vi "Main Abstraction Level 6.vi"() -> ()   [LabVIEW 2023]
doc: "This is the complete measurement application, the result of all the design effort in the earlier Main Abstraction Level VIs."
uses:
  subVIs/Simulated Signal Type.ctl
  messages/MeasureAndLogMessage.lvclass/MeasureAndLogMessage.ctl
  subVIs/Measure and Log Settings.ctl
  <extravilib>/ChannelInstances/Stream-a[.](wfm(dbl))/EndpointRead.vi
  <vilib>/ChannelSupport/Channel Message/Read ID.vi
  <extravilib>/ChannelInstances/Stream-a[.](wfm(dbl))/Endpoint.vi
  <extravilib>/ChannelInstances/Stream-str/EndpointRead.vi
  <extravilib>/ChannelInstances/Lossy Stream-a[.](wfm(dbl))/EndpointRead.vi
  <extravilib>/ChannelInstances/Lossy Stream-a[.](wfm(dbl))/Endpoint.vi
  <extravilib>/ChannelInstances/Stream-str/Endpoint.vi
  messages/MeasureAndLogMessage.lvclass
  c:/dev/_r/4/eng/lv-core/lvpostprocessingd/lv_mc_x86_64/dist_i386/vi.lib/ChannelSupport/Channel Message/Channel Message.lvclass
  <extravilib>/ChannelInstances/Tag-path/Instantiate.vi
  <extravilib>/ChannelInstances/Stream-a[.](wfm(dbl))/Instantiate.vi
  <extravilib>/ChannelInstances/Stream-a[.](wfm(dbl))/)Channel.vi
  <resource>/ChannelSupport/_ChannelSupport/WaitIfNeeded.vi
  <extravilib>/ChannelInstances/Tag-path/EndpointRead.vi
  <vilib>/Waveform/WDTFileIO.llb/Write Waveforms to File (1D).vi
  <extravilib>/ChannelInstances/Lossy Stream-a[.](wfm(dbl))/Instantiate.vi
  <extravilib>/ChannelInstances/Lossy Stream-a[.](wfm(dbl))/)Channel.vi
  <extravilib>/ChannelInstances/Messenger-class'MeasureAndLogMessage'/Instantiate.vi
  <extravilib>/ChannelInstances/Messenger-class'MeasureAndLogMessage'/Endpoint.vi
  <extravilib>/ChannelInstances/Stream-str/Instantiate.vi
  <extravilib>/ChannelInstances/Stream-str/)Channel.vi
  <extravilib>/ChannelInstances/Tag-bool/Instantiate.vi
  <extravilib>/ChannelInstances/Tag-t'Measure and Log Settings.ctl'/Instantiate.vi
  <extravilib>/ChannelInstances/Tag-t'Measure and Log Settings.ctl'/Endpoint.vi
  <extravilib>/ChannelInstances/Tag-path/Endpoint.vi
  <extravilib>/ChannelInstances/Tag-bool/Endpoint.vi
  <extravilib>/ChannelInstances/Tag-bool/EndpointRead.vi
  <extravilib>/ChannelInstances/Tag-t'Measure and Log Settings.ctl'/EndpointRead.vi
  <extravilib>/ChannelInstances/Stream-str.lvlib
  <extravilib>/ChannelInstances/Lossy Stream-a[.](wfm(dbl)).lvlib
  <extravilib>/ChannelInstances/Tag-bool.lvlib
  <extravilib>/ChannelInstances/Stream-a[.](wfm(dbl)).lvlib
  <extravilib>/ChannelInstances/Tag-path.lvlib
  <extravilib>/ChannelInstances/Tag-t'Measure and Log Settings.ctl'.lvlib
  <extravilib>/ChannelInstances/Messenger-class'MeasureAndLogMessage'.lvlib
panel:
  in  "Exit flag":bool
  in  "Record":bool
  in  "Stop":bool
  out "Data":waveform(dbl)[](graph)
  out "Status":string
  in  "Settings":bool
  in  "Start":bool
  in  "Exit":bool
  # "Continuous Measurement Data Logger"
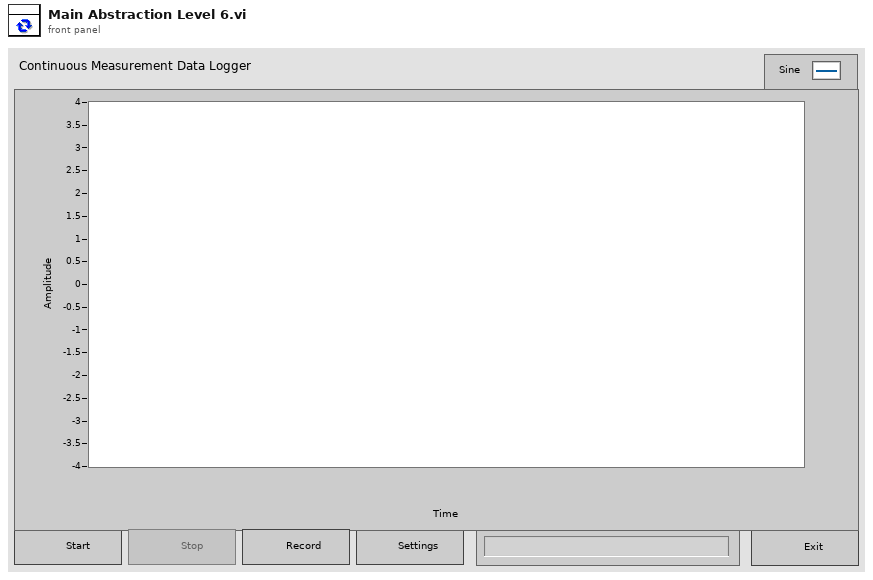
[diagram p1: front panel]
types:
  T1 = typedef "Measure and Log Settings.ctl" = cluster{"sample rate":dbl, "input range":dbl, "logfile path":path, "Simulated Signal":cluster{"signal type":T2, "frequency":dbl, "amplitude":dbl}}
  T2 = typedef "Simulated Signal Type.ctl" = enum16{"Sine Wave", "Square Wave with Noise"}
  T3 = enum8{"Enabled", "Disabled", "Disabled and Grayed Out"}
  T4 = typedef "Messenger-class'MeasureAndLogMessage'.lvlib/))Channel.ctl" = refnum<queue>
  T5 = typedef "Tag-t'Measure and Log Settings.ctl'.lvlib/))Channel.ctl" = refnum<queue>
  T6 = typedef "Tag-path.lvlib/))Channel.ctl" = refnum<queue>
  T7 = typedef "Tag-bool.lvlib/))Channel.ctl" = refnum<queue>
  T8 = typedef "Stream-a[.](wfm(dbl)).lvlib/)Channel.ctl" = refnum<queue>
  T9 = typedef "Stream-str.lvlib/)Channel.ctl" = refnum<queue>
  T10 = typedef "Lossy Stream-a[.](wfm(dbl)).lvlib/)Channel.ctl" = refnum<queue>
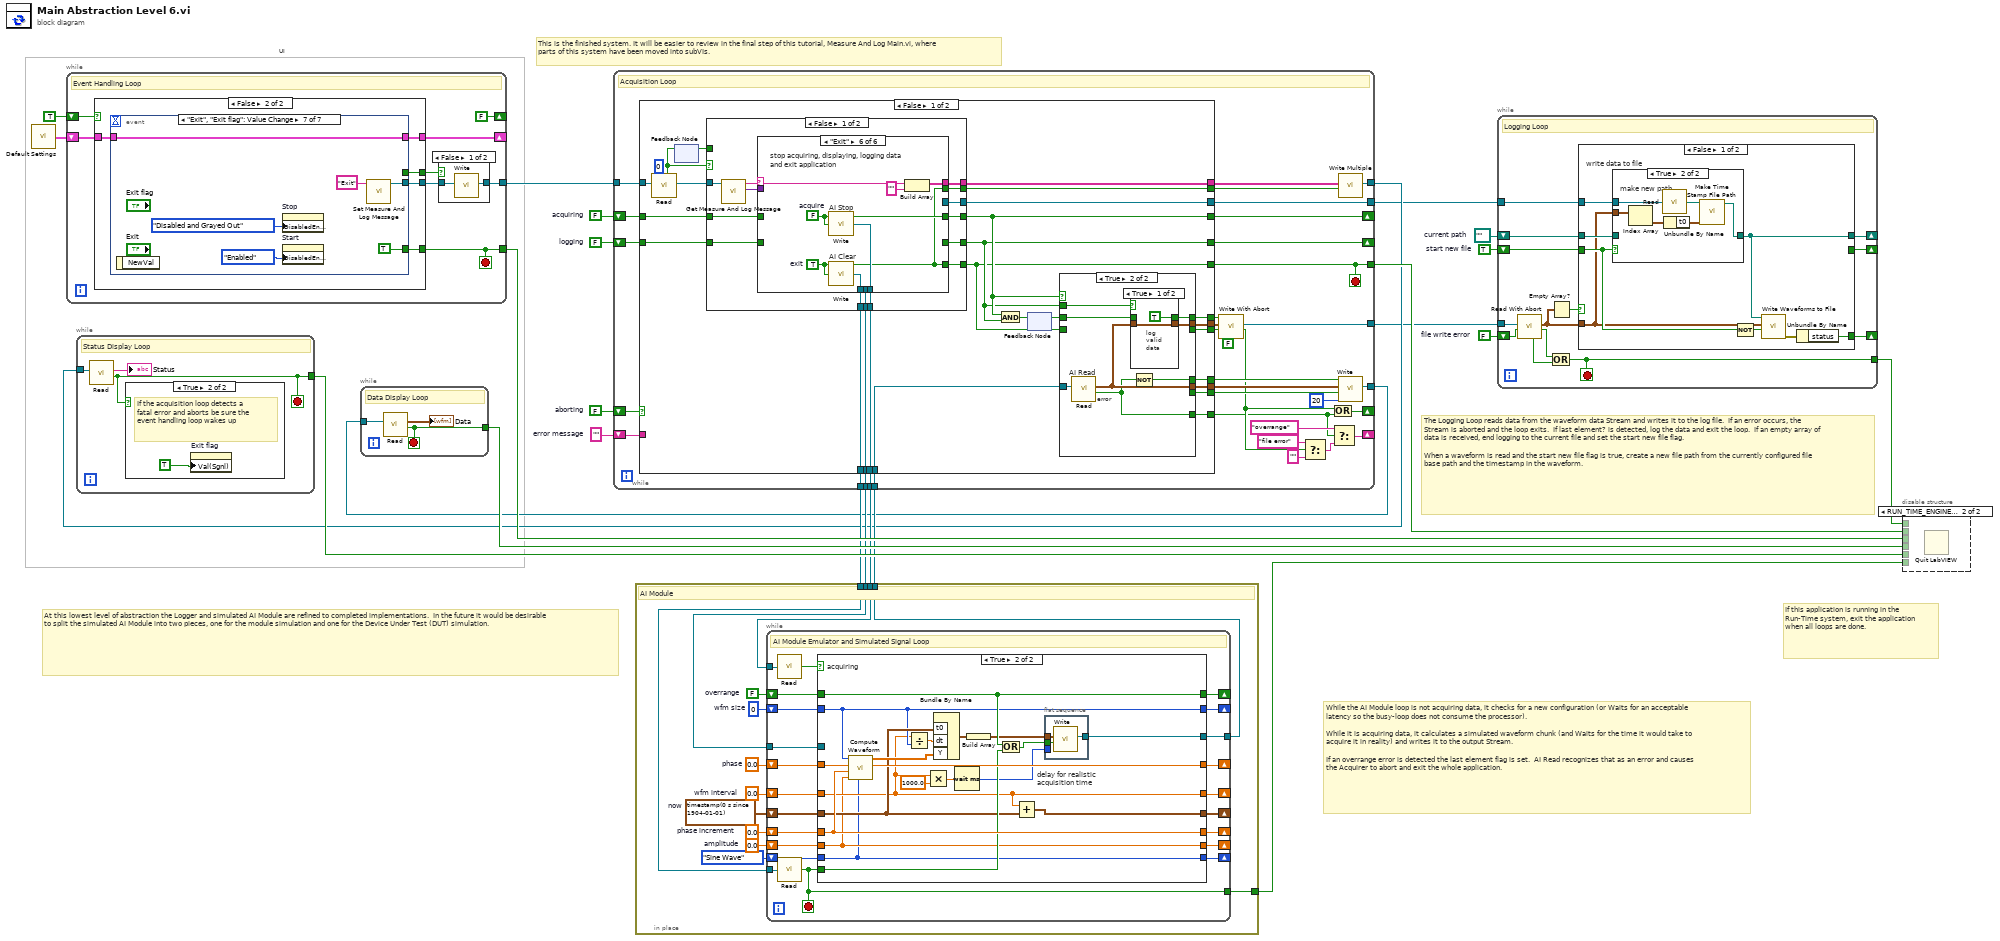
[diagram p0: block diagram]
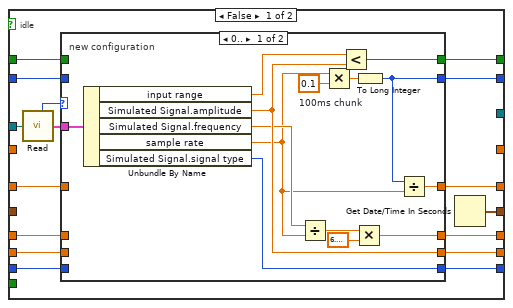
[diagram p2: hidden frame]
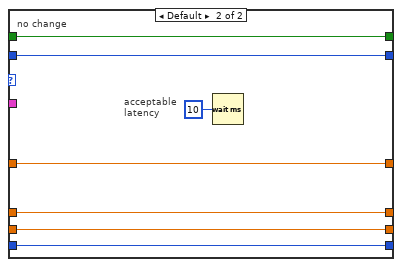
[diagram p3: hidden frame]
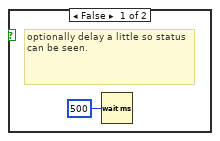
[diagram p4: hidden frame]
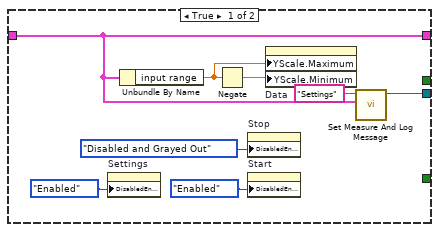
[diagram p5: hidden frame]
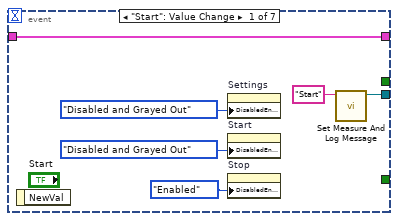
[diagram p6: hidden frame]
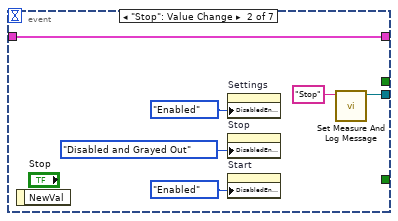
[diagram p7: hidden frame]
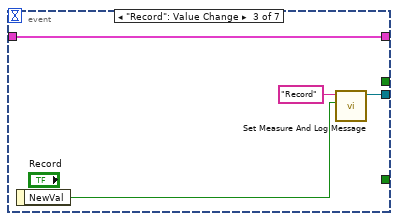
[diagram p8: hidden frame]
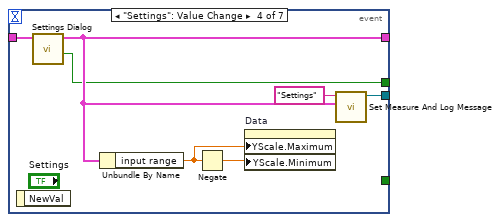
[diagram p9: hidden frame]
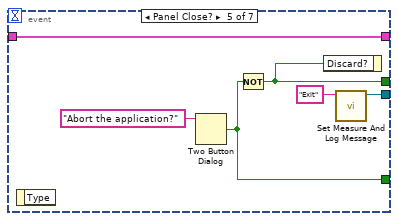
[diagram p10: hidden frame]
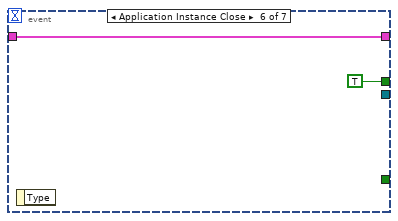
[diagram p11: hidden frame]
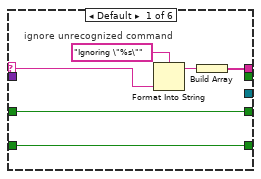
[diagram p14: hidden frame]
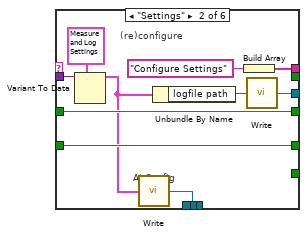
[diagram p15: hidden frame]
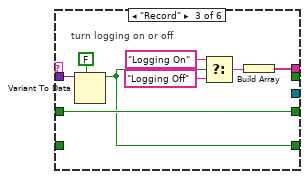
[diagram p16: hidden frame]
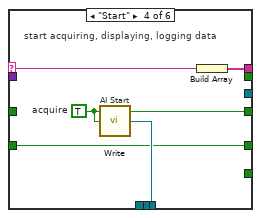
[diagram p17: hidden frame]
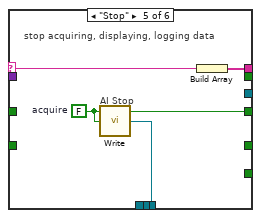
[diagram p18: hidden frame]
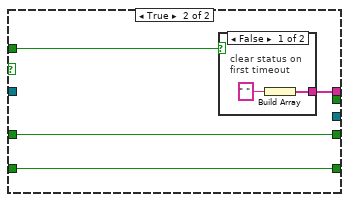
[diagram p19: hidden frame]
diagram:
  w2 = ""  # error message
  w4 = FALSE  # file write error
  w5 = path ""  # current path
  w6 = TRUE  # start new file
  w8 = FALSE  # aborting
  w10 = FALSE  # logging
  w11 = FALSE  # acquiring
  # "This is the finished system. It will be easier to review in the final step of this tutorial, Measure And Log Main.vi, where parts of this system have been moved into subVIs."
  # "At this lowest level of abstraction the Logger and simulated AI Module are refined to completed implementations.  In the future it would be desirable to split the simulated AI Module into two pieces, one for the module simulation and one for the Device Under Test (DUT) simulation."
  # "If this application is running in the Run-Time system, exit the application when all loops are done."
  # "The Logging Loop reads data from the waveform data Stream and writes it to the log file.  If an error occurs, the Stream is aborted and the loop exits.  If last element? is detected, log the data and exit the loop.  If an empty array of data is received, end logging to the current file and set the start new file flag.\n\nWhen a waveform is read and the start new file flag is true, create a new file path from the currently configured file base path and the timestamp in the waveform."
  # "While the AI Module loop is not acquiring data, it checks for a new configuration (or Waits for an acceptable latency so the busy-loop does not consume the processor).\n\nWhile it is acquiring data, it calculates a simulated waveform chunk (and Waits for the time it would take to acquire it in reality) and writes it to the output Stream.\n\nIf an overrange error is detected the last element flag is set.  AI Read recognizes that as an error and causes the Acquirer to abort and exit the whole application."
  # "UI"
  n1 = call "Default Settings.vi"() -> ("default settings"=w7:T1)
  n2 = while {
    tunnel: [w29] -> w14
    tunnel: [w32] -> w24
    shift-right: [w31] -> _
    shift-left: w7 -> [w30]
    shift-right: [FALSE] -> _
    shift-left: TRUE -> [w26]
    stop <- w32 stop-if-true
    # "Event Handling Loop"
    n3 = case shown="False" w26 {
      tunnel: [_ w45] -> w32
      tunnel: [w39 w44] -> w31
      tunnel: w30 -> [w39 w43]
      tunnel: [w35 w42] -> w28
      tunnel: [_ w41] -> w27
      frame True {
        n4 = property on="Settings" class="Bool"("DisabledEnum"=T3."Enabled" ("Disabled")) -> ()  [unwired: 2 in, 2 out]
        n5 = Unbundle By Name(w39) -> ("input range"=w33:dbl)
        n6 = Negate(x=w33) -> (-x=w34:dbl)
        n7 = property on="Stop" class="Bool"("DisabledEnum"=T3."Disabled and Grayed Out" ("Disabled")) -> ()  [unwired: 2 in, 2 out]
        n8 = property on="Start" class="Bool"("DisabledEnum"=T3."Enabled" ("Disabled")) -> ()  [unwired: 2 in, 2 out]
        n9 = property on="Data" class="WFChart (strict)"("YScale.Maximum"=w33, "YScale.Minimum"=w34) -> ()  [unwired: 2 in, 2 out]
        n10 = call "Set Measure And Log Message.vi"("args"=w39, "command"="Settings") -> ("MyMessage"=w35:refnum<class "MeasureAndLogMessage.lvclass">)  [unwired: 9 in]
      }
      frame False {
        n11 = event shown="[6] \"Exit\", \"Exit flag\": Value Change" {
          selector: _ -> [_ _ _ _ _ _ _]
          dyn-events: _ -> [_ _ _ _ _ _ _]
          timeout: _ -> [_ _ _ _ _ _ _]
          tunnel: [_ _ _ _ w70 _ TRUE] -> w45
          tunnel: [w47 w53 w59 w67 w73 w76 w78] -> w44
          tunnel: w43 -> [w47 w53 w59 w68 w73 w76 w78]
          tunnel: [w46 w52 w58 w66 w71 _ w77] -> w42
          tunnel: [_ _ _ w64 w69 TRUE ("cancelled") _] -> w41
          event "Start": Value Change {
            n12 = event-data() -> ()  [unwired: 1 in, 1 out]
            n13 = property on="Settings" class="Bool"("DisabledEnum"=T3."Disabled and Grayed Out" ("Disabled")) -> ()  [unwired: 2 in, 2 out]
            n14 = property on="Start" class="Bool"("DisabledEnum"=T3."Disabled and Grayed Out" ("Disabled")) -> ()  [unwired: 2 in, 2 out]
            n15 = property on="Stop" class="Bool"("DisabledEnum"=T3."Enabled" ("Disabled")) -> ()  [unwired: 2 in, 2 out]
            n16 = call "Set Measure And Log Message.vi"("command"="Start") -> ("MyMessage"=w46:refnum<class "MeasureAndLogMessage.lvclass">)  [unwired: 10 in]
          }
          event "Stop": Value Change {
            n17 = event-data() -> ()  [unwired: 1 in, 1 out]
            n18 = property on="Settings" class="Bool"("DisabledEnum"=T3."Enabled" ("Disabled")) -> ()  [unwired: 2 in, 2 out]
            n19 = property on="Stop" class="Bool"("DisabledEnum"=T3."Disabled and Grayed Out" ("Disabled")) -> ()  [unwired: 2 in, 2 out]
            n20 = property on="Start" class="Bool"("DisabledEnum"=T3."Enabled" ("Disabled")) -> ()  [unwired: 2 in, 2 out]
            n21 = call "Set Measure And Log Message.vi"("command"="Stop") -> ("MyMessage"=w52:refnum<class "MeasureAndLogMessage.lvclass">)  [unwired: 10 in]
          }
          event "Record": Value Change {
            n22 = event-data() -> ("NewVal"=w60:bool)  [unwired: 1 in]
            n23 = call "Set Measure And Log Message.vi"("args"=w60, "command"="Record") -> ("MyMessage"=w58:refnum<class "MeasureAndLogMessage.lvclass">)  [unwired: 9 in]
          }
          event "Settings": Value Change {
            n24 = event-data() -> ()  [unwired: 1 in, 1 out]
            n25 = call "Settings Dialog.vi"("settings in"=w68) -> ("cancelled"=w64:bool, "settings out"=w67:T1)  [unwired: 9 in]
            n26 = Unbundle By Name(w67) -> ("input range"=w62:dbl)
            n27 = Negate(x=w62) -> (-x=w63:dbl)
            n28 = property on="Data" class="WFChart (strict)"("YScale.Maximum"=w62, "YScale.Minimum"=w63) -> ()  [unwired: 2 in, 2 out]
            n29 = call "Set Measure And Log Message.vi"("args"=w67, "command"="Settings") -> ("MyMessage"=w66:refnum<class "MeasureAndLogMessage.lvclass">)  [unwired: 9 in]
          }
          event Panel Close? {
            n30 = event-data() -> ()  [unwired: 1 in, 1 out]
            n31 = Two Button Dialog(message="Abort the application?") -> (T button?=w70:bool)  [unwired: 2 in]
            n32 = Not(x=w70) -> (.not. x?=w69:bool)
            n33 = event-data("Discard?"=w69) -> ()  [unwired: 1 in, 1 out]
            n34 = call "Set Measure And Log Message.vi"("command"="Exit") -> ("MyMessage"=w71:refnum<class "MeasureAndLogMessage.lvclass">)  [unwired: 10 in]
          }
          event Application Instance Close {
            n35 = event-data() -> ()  [unwired: 1 in, 1 out]
          }
          event "Exit", "Exit flag": Value Change {
            n36 = event-data() -> ()  [unwired: 1 in, 1 out]
            n37 = property on="Stop" class="Bool"("DisabledEnum"=T3."Disabled and Grayed Out" ("Disabled")) -> ()  [unwired: 2 in, 2 out]
            n38 = property on="Start" class="Bool"("DisabledEnum"=T3."Enabled" ("Disabled")) -> ()  [unwired: 2 in, 2 out]
            n39 = call "Set Measure And Log Message.vi"("command"="Exit") -> ("MyMessage"=w77:refnum<class "MeasureAndLogMessage.lvclass">)  [unwired: 10 in]
          }
        }
      }
    }
    n40 = case shown="False" w27 {
      tunnel: [w84 _] -> w29
      tunnel: w28 -> [w83 _]
      frame False {
        n41 = call <extravilib>:"Write.vi"("element"=w83) -> ("channel"=w84:T4)  [unwired: 8 in, 2 out]
      }
      frame True {
      }
    }
  }
  n42 = while {
    tunnel: w15 -> [w87]
    tunnel: [w85] -> w23
    stop <- w85 stop-if-true
    # "Status Display Loop"
    n43 = call <extravilib>:"Read.vi"("channel"=w87) -> ("last element?"=w85:bool, "element"=→"Status":string)  [unwired: 6 in, 3 out]
    n44 = case shown="True" w85 {
      frame False {
        # "optionally delay a little so status can be seen."
        n45 = Wait (ms)(milliseconds to wait=u32 500) -> ()  [unwired: 1 out]
      }
      frame True {
        # "If the acquisition loop detects a fatal error and aborts be sure the event handling loop wakes up"
        n46 = property on="Exit flag" class="Bool (strict)"("Val(Sgnl)"=TRUE) -> ()  [unwired: 2 in, 2 out]
      }
    }
  }
  n47 = while {
    tunnel: [w92] -> w22
    tunnel: w13 -> [w90]
    stop <- w92 stop-if-true
    # "Data Display Loop"
    n48 = call <extravilib>:"Read.vi"("channel"=w90) -> ("last element?"=w92:bool, "element"=→"Data":waveform(dbl)[])  [unwired: 5 in, 4 out]
  }
  n49 = while {
    tunnel: w14 -> [w125]
    tunnel: [w113] -> w15
    tunnel: [w110] -> w13
    tunnel: [w106] -> w12
    tunnel: [w121] -> w18
    tunnel: w19 -> [w124]
    shift-right: [w118] -> _
    shift-left: w11 -> [w119]
    shift-right: [w117] -> _
    shift-left: w10 -> [w126]
    tunnel: [w123] -> w9
    tunnel: [w122] -> w17
    tunnel: [w120] -> w16
    shift-right: [w105] -> _
    shift-left: w8 -> [w116]
    shift-right: [w96] -> _
    shift-left: w2 -> [w115]
    tunnel: [w114] -> w21
    stop <- w114 stop-if-true
    # "Acquisition Loop"
    n50 = case shown="False" w116 {
      tunnel: w126 -> [w152 _]
      tunnel: w125 -> [w151 _]
      tunnel: w124 -> [w149 _]
      tunnel: [w145 _] -> w123
      tunnel: [w144 _] -> w122
      tunnel: [w143 w231] -> w121
      tunnel: [w142 w230] -> w120
      tunnel: w119 -> [w141 _]
      tunnel: [w140 w232] -> w118
      tunnel: [w139 _] -> w117
      tunnel: [w136 w227] -> w114
      tunnel: w115 -> [_ w229]
      tunnel: [w134 w227] -> w112
      tunnel: [w135 w228] -> w111
      tunnel: [w132 w227] -> w109
      tunnel: [w133 _] -> w108
      tunnel: [w131 _] -> w107
      tunnel: [w130 _] -> w97
      tunnel: [w129 _] -> w104
      tunnel: [w128 w227] -> w103
      tunnel: [w127 _] -> w102
      frame False {
        n51 = call <extravilib>:"Read.vi"("timeout in ms (-1)"=0, "channel"=w151) -> ("element"=w150:refnum<class "MeasureAndLogMessage.lvclass">, "timed out?"=w147:bool)  [unwired: 7 in, 1 out]
        n52 = feedback #1() -> (w146:bool)  [unwired: 1 in]
        n53 = feedback-in #1(w147) -> ()
        n54 = case shown="False" w147 {
          tunnel: w150 -> [w166 _]
          tunnel: [w162 _] -> w143
          tunnel: [w163 _] -> w136
          tunnel: [w161 w210] -> w140
          tunnel: w141 -> [w160 w210]
          tunnel: [w159 w209] -> w139
          tunnel: w152 -> [w158 w209]
          tunnel: w146 -> [_ w208]
          tunnel: [w157 _] -> w145
          tunnel: [w156 _] -> w144
          tunnel: [w155 _] -> w142
          tunnel: [w154 w207] -> w135
          tunnel: [w153 _] -> w134
          frame False {
            n55 = call "Get Measure And Log Message.vi"("MyMessage"=w166) -> ("args"=w164:variant, "command"=w165:string)  [unwired: 7 in, 2 out]
            n56 = case shown="\"Exit\"" w165 {
              selector: w165 -> [w172 _ _ w192 w197 w206]
              tunnel: w164 -> [_ w180 w189 _ _ _]
              tunnel: [_ _ _ w195 w199 w203] -> w162
              tunnel: [_ _ _ _ _ w200] -> w163
              tunnel: [w170 w182 w190 w194 w198 w204] -> w161
              tunnel: w160 -> [w170 w182 w190 _ _ _]
              tunnel: [w169 w181 w185 w193 _ _] -> w159
              tunnel: w158 -> [w169 w181 _ w193 _ _]
              tunnel: [_ w177 _ _ _ _] -> w157
              tunnel: [_ w176 _ _ _ _] -> w156
              tunnel: [_ _ _ _ _ w202] -> w155
              tunnel: [w167 w173 w183 w191 w196 w201] -> w154
              tunnel: [_ _ _ _ _ w200] -> w153
              frame Default {
                # "ignore unrecognized command"
                n57 = Format Into String(format string="Ignoring \"%s\"", w172) -> (resulting string=w168:string)  [unwired: 2 in, 1 out]
                n58 = Build Array(w168) -> (w167:string[])
              }
              frame "Settings" {
                # "AI Config"
                # "(re)configure"
                n59 = Variant To Data(type=T1 {"sample rate"=100.0, "input range"=10.0, "logfile path"=path "/Bohr/Users/jeffk/Documents/LabVIEW Data/Logged Data.tdms", "Simulated Signal"={"signal type"=enum."Sine Wave", "frequency"=1000.0, "amplitude"=5.0}} ("settings out"), Variant=w180) -> (data=w179:T1)  [unwired: 1 in, 1 out]
                n60 = call <extravilib>:"Write.vi"("element"=w179) -> ("channel"=w176:T5)  [unwired: 1 out]
                n61 = Unbundle By Name(w179) -> ("logfile path"=w178:path)
                n62 = Build Array("Configure Settings" ("element")) -> (w173:string[])
                n63 = call <extravilib>:"Write.vi"("element"=w178) -> ("channel"=w177:T6)  [unwired: 1 out]
              }
              frame "Record" {
                # "turn logging on or off"
                n64 = Variant To Data(type=FALSE, Variant=w189) -> (data=w185:bool)  [unwired: 1 in, 1 out]
                n65 = Select(t="Logging On", s=w185, f="Logging Off") -> (s? t:f=w184:string)
                n66 = Build Array(w184) -> (w183:string[])
              }
              frame "Start" {
                w194 = TRUE  # acquire
                # "AI Start"
                # "start acquiring, displaying, logging data"
                n67 = call <extravilib>:"Write.vi"("element"=w194) -> ("channel"=w195:T7)  [unwired: 1 out]
                n68 = Build Array(w192) -> (w191:string[])
              }
              frame "Stop" {
                w198 = FALSE  # acquire
                # "AI Stop"
                # "stop acquiring, displaying, logging data"
                n69 = call <extravilib>:"Write.vi"("element"=w198) -> ("channel"=w199:T7)  [unwired: 1 out]
                n70 = Build Array(w197) -> (w196:string[])
              }
              frame "Exit" {
                w204 = FALSE  # acquire
                w200 = TRUE  # exit
                # "AI Clear"
                # "AI Stop"
                # "stop acquiring, displaying, logging data\nand exit application"
                n71 = call <extravilib>:"Write.vi"("element"=w204) -> ("channel"=w203:T7)  [unwired: 1 out]
                n72 = call <extravilib>:"Write.vi"("element"=w200) -> ("channel"=w202:T7)  [unwired: 1 out]
                n73 = Build Array(w206, "" ("element")) -> (w201:string[])
              }
            }
          }
          frame True {
            n74 = case shown="False" w208 {
              tunnel: [w211 _] -> w207
              frame False {
                # "clear status on\nfirst timeout"
                n75 = Build Array(" " ("string")) -> (w211:string[])
              }
              frame True {
              }
            }
          }
        }
        n76 = And(x=w140, y=w139) -> (x .and. y?=w138:bool)
        n77 = feedback #2() -> (w137:bool)  [unwired: 1 in]
        n78 = feedback-in #2(w138) -> ()
        n79 = case shown="True" w140 {
          tunnel: w149 -> [_ w223]
          tunnel: w139 -> [_ w222]
          tunnel: w137 -> [w215 w221]
          tunnel: w136 -> [w214 _]
          tunnel: [_ w219] -> w133
          tunnel: [w214 _] -> w132
          tunnel: [_ w220] -> w131
          tunnel: [_ w216] -> w130
          tunnel: [w215 w217] -> w129
          tunnel: [w214 _] -> w128
          tunnel: [_ w218] -> w127
          frame False {
            # "acceptable\nlatency"
            n80 = Wait (ms)(milliseconds to wait=u32 30) -> ()  [unwired: 1 out]
          }
          frame True {
            # "error"
            # "AI Read"
            n81 = call <extravilib>:"Read.vi"("channel"=w223) -> ("last element?"=w216:bool, "element"=w220:waveform(dbl)[])  [unwired: 6 in, 3 out]
            n82 = case shown="True" w222 {
              tunnel: w220 -> [w225 _]
              tunnel: w221 -> [_ w226]
              tunnel: [w225 _] -> w218
              tunnel: [TRUE w226] -> w217
              frame True {
                # "log \nvalid\ndata"
              }
              frame False {
              }
            }
            n83 = Not(x=w216) -> (.not. x?=w219:bool)
          }
        }
      }
      frame True {
        w232 = FALSE  # acquire
        w227 = TRUE  # exit
        # "aborting due to AI or file error"
        # "AI Clear"
        # "AI Stop"
        # "stop acquiring, displaying, logging data\nand exit application with error message"
        n84 = call <extravilib>:"Write.vi"("element"=w232) -> ("channel"=w231:T7)  [unwired: 1 out]
        n85 = call <extravilib>:"Write.vi"("element"=w227) -> ("channel"=w230:T7)  [unwired: 1 out]
        n86 = Build Array(w229) -> (w228:string[])
      }
    }
    n87 = call <extravilib>:"Write With Abort.vi"("abort"=FALSE, "last element? (F)"=w103, "element"=w102, "element valid? (T)"=w104) -> ("aborted?"=w100:bool, "channel"=w106:T8)  [unwired: 4 in, 2 out]
    n88 = Select(t="file error", s=w100, f="") -> (s? t:f=w95:string)
    n89 = Or(x=w100, y=w97) -> (x .or. y?=w105:bool)
    n90 = Select(t="overrange", s=w97, f=w95) -> (s? t:f=w96:string)
    n91 = call <extravilib>:"Write Multiple.vi"("last element? (F)"=w112, "elements"=w111) -> ("channel"=w113:T9)  [unwired: 6 in, 3 out]
    n92 = call <extravilib>:"Write.vi"("size (1)"=20, "last element? (F)"=w109, "element"=w107, "element valid? (T)"=w108) -> ("channel"=w110:T10)  [unwired: 5 in, 2 out]
  }
  n93 = in-place {
    in-place-border: [w243] -> w19
    in-place-border: w18 -> [w242]
    in-place-border: w17 -> [w241]
    in-place-border: w16 -> [w240]
    in-place-border: [w233] -> w20
    w235 = timestamp(0 s since 1904-01-01)  # now
    w236 = 0.0  # wfm interval
    w237 = 0  # wfm size
    w238 = FALSE  # overrange
    w239 = 0.0  # amplitude
    w245 = 0.0  # phase increment
    w244 = 0.0  # phase
    # "AI Module"
    n94 = while {
      shift-right: [w266] -> _
      shift-left: w244 -> [w267]
      tunnel: [w265] -> w243
      tunnel: w242 -> [w262]
      tunnel: w240 -> [w261]
      tunnel: w241 -> [w260]
      shift-right: [w259] -> _
      shift-left: w245 -> [w264]
      shift-right: [w258] -> _
      shift-left: Simulated_Signal_Type."Sine Wave" ("signal type") -> [w257]
      shift-right: [w256] -> _
      shift-left: w239 -> [w255]
      shift-right: [w254] -> _
      shift-left: w238 -> [w253]
      shift-right: [w252] -> _
      shift-left: w237 -> [w251]
      shift-right: [w250] -> _
      shift-left: w236 -> [w248]
      shift-right: [w249] -> _
      shift-left: w235 -> [w247]
      tunnel: [w246] -> w233
      stop <- w246 stop-if-true
      # "AI Module Emulator and Simulated Signal Loop"
      n95 = call <extravilib>:"Read.vi"("channel"=w262) -> ("element"=w263:bool)  [unwired: 1 in, 1 out]
      n96 = call <extravilib>:"Read.vi"("channel"=w261) -> ("element"=w246:bool)  [unwired: 1 in, 1 out]
      n97 = case shown="True" w263 {
        tunnel: w267 -> [_ w324]
        tunnel: [_ w323] -> w266
        tunnel: [_ w312] -> w265
        tunnel: w264 -> [w283 w322]
        tunnel: w246 -> [_ w320]
        tunnel: w260 -> [w270 _]
        tunnel: [w282 w322] -> w259
        tunnel: [w281 w306] -> w258
        tunnel: w257 -> [w280 w306]
        tunnel: [w279 w307] -> w256
        tunnel: w255 -> [w278 w307]
        tunnel: [w277 w321] -> w254
        tunnel: w253 -> [w276 w321]
        tunnel: [w275 w315] -> w252
        tunnel: w251 -> [w274 w315]
        tunnel: [w273 w311] -> w250
        tunnel: [w272 w319] -> w249
        tunnel: w248 -> [w271 w311]
        tunnel: w247 -> [_ w317]
        frame False {
          # "idle"
          n98 = call <extravilib>:"Read.vi"("channel"=w270) -> ("missed"=w269:i32, "element"=w268:T1)  [unwired: 1 in]
          n99 = case shown="0.." w269 {
            tunnel: w268 -> [w297 _]
            tunnel: w283 -> [_ w304]
            tunnel: [w290 w304] -> w282
            tunnel: [w295 w303] -> w281
            tunnel: w280 -> [_ w303]
            tunnel: [w292 w302] -> w279
            tunnel: w278 -> [_ w302]
            tunnel: [w294 w301] -> w277
            tunnel: w276 -> [_ w301]
            tunnel: [w286 w300] -> w275
            tunnel: w274 -> [_ w300]
            tunnel: [w285 w299] -> w273
            tunnel: w271 -> [_ w299]
            frame 0.. {
              w289 = 0.1  # 100ms chunk
              # "new configuration"
              n100 = Unbundle By Name(w297) -> ("input range"=w293:dbl, "Simulated Signal.amplitude"=w292:dbl, "Simulated Signal.frequency"=w287:dbl, "sample rate"=w284:dbl, "Simulated Signal.signal type"=w295:T2)
              n101 = Divide(x=w287, y=w284) -> (x/y=w291:dbl)
              n102 = Multiply(x=w284, y=w289) -> (x*y=w288:dbl)
              n103 = Less?(x=w293, y=w292) -> (x < y?=w294:bool)
              n104 = Multiply(x=w291, y=6.283185307179586) -> (x*y=w290:dbl)
              n105 = To Long Integer(number=w288) -> (32bit integer=w286:i32)
              n106 = Divide(x=w286, y=w284) -> (x/y=w285:dbl)
            }
            frame Default {
              # "acceptable\nlatency"
              # "no change"
              n107 = Wait (ms)(milliseconds to wait=u32 10) -> ()  [unwired: 1 out]
            }
          }
          n108 = Get Date/Time In Seconds() -> (seconds since 1Jan1904=w272:timestamp)
        }
        frame True {
          # "delay for realistic\nacquisition time"
          # "acquiring"
          n109 = call "Compute Waveform.vi"("signal type"=w306, "amplitude"=w307, "phase increment"=w322, "phase in"=w324, "wfm size"=w315) -> ("phase out"=w323:dbl, "wfm array"=w318:dbl[])  [unwired: 5 in]
          n110 = Divide(x=w311, y=w315) -> (x/y=w316:dbl)
          n111 = Multiply(x=w311, y=1000.0) -> (x*y=w309:dbl)
          n112 = Bundle By Name("t0"=w317, "dt"=w316, "Y"=w318) -> (w314:waveform(dbl))  [unwired: 1 in]
          n113 = Wait (ms)(milliseconds to wait=w309) -> (millisecond timer value=w305:u32)
          n114 = Build Array(w314) -> (w313:waveform(dbl)[])
          n115 = Or(x=w321, y=w320) -> (x .or. y?=w308:bool)
          n116 = Add(x=w311, y=w317) -> (x+y=w319:timestamp)
          n117 = flat-sequence {
            tunnel: w313 -> [w327]
            tunnel: [w326] -> w312
            tunnel: w308 -> [w325]
            tunnel: w305 -> [_]
            frame #0 {
              n118 = call <extravilib>:"Write.vi"("last element? (F)"=w325, "element"=w327) -> ("channel"=w326:T8)  [unwired: 7 in, 2 out]
            }
          }
        }
      }
    }
  }
  n119 = while {
    tunnel: w12 -> [w340]
    tunnel: w9 -> [w335]
    shift-right: [w337] -> _
    shift-left: w6 -> [w336]
    shift-right: [w334] -> _
    shift-left: w5 -> [w333]
    shift-right: [w331] -> _
    shift-left: w4 -> [w330]
    tunnel: [w328] -> w3
    stop <- w328 stop-if-true
    # "Logging Loop"
    n120 = call <extravilib>:"Read With Abort.vi"("abort"=w330, "channel"=w340) -> ("last element?"=w338:bool, "element"=w339:waveform(dbl)[], "aborted?"=w329:bool)  [unwired: 4 in, 3 out]
    n121 = Or(x=w338, y=w329) -> (x .or. y?=w328:bool)
    n122 = Empty Array?(array=w339) -> (empty?=w332:bool)
    n123 = case shown="False" w332 {
      selector: w332 -> [_ w356]
      tunnel: w339 -> [w343 _]
      tunnel: [_ w356] -> w337
      tunnel: w336 -> [w344 _]
      tunnel: w335 -> [w347 _]
      tunnel: [w345 _] -> w334
      tunnel: w333 -> [w346 _]
      tunnel: [w341 _] -> w331
      frame False {
        # "write data to file"
        n124 = case shown="True" w344 {
          tunnel: w347 -> [_ w355]
          tunnel: w343 -> [_ w352]
          tunnel: [w349 w354] -> w345
          tunnel: w346 -> [w349 _]
          frame False {
          }
          frame True {
            # "make new path"
            n125 = Index Array(array=w352) -> (element=w353:waveform(dbl))  [unwired: 1 in]
            n126 = call <extravilib>:"Read.vi"("channel"=w355) -> ("element"=w351:path)  [unwired: 1 in, 1 out]
            n127 = Unbundle By Name(w353) -> ("t0"=w350:timestamp)
            n128 = call "Make Time Stamp File Path.vi"("t0"=w350, "base path"=w351) -> ("file path"=w354:path)  [unwired: 9 in]
          }
        }
        n129 = Not(x=w344) -> (.not. x?=w348:bool)
        n130 = call-poly <vilib>:"Write Waveforms to File.vi"("append to file? (new file:F)"=w348, "waveform array"=w343, "file path (dialog if empty)"=w345) -> ("error out"=w342:errorcluster)  [unwired: 7 in, 1 out]
        n131 = Unbundle By Name(w342) -> ("status"=w341:bool)
      }
      frame True {
        # "empty: start new file next time"
      }
    }
  }
  n132 = disable-structure shown="RUN_TIME_ENGINE==True" {
    disable-tunnel: w24 -> [_ _]
    disable-tunnel: w23 -> [_ _]
    disable-tunnel: w22 -> [_ _]
    disable-tunnel: w20 -> [_ _]
    disable-tunnel: w3 -> [_ _]
    disable-tunnel: w21 -> [_ _]
    frame condition #0 (active) {
    }
    frame condition #1 {
      n133 = Quit LabVIEW() -> ()  [unwired: 1 in]
    }
  }
